vi "Control.vi"(4 "vB":fxp<+,28,8>, 5 "vB_o":fxp<+,28,8>, 6 "Vb":fxp<+,27,7>, 7 "e(k-1)":fxp<+/-,29,9>, 8 "s_c":bool, 9 "Io":fxp<+/-,25,5>, 10 "u(k-1)":fxp<+,20,0>, 11 "v_ref":fxp<+,28,8>) -> (2 "u(k)":fxp<+,20,0>, 3 "e(k)":fxp<+/-,29,9>)   [LabVIEW 2015]
uses:
  <vilib>/rvi/FXPMathLib/FxpMul/XNode/nifxpmath_Multiplier.xnode
  <vilib>/rvi/FXPMathLib/FxpSub/XNode/nifxpmath_Sub.xnode
  <vilib>/rvi/FXPMathLib/FxpAdd/XNode/nifxpmath_Add.xnode
  <vilib>/rvi/FXPMathLib/sim/FxpSim.dll
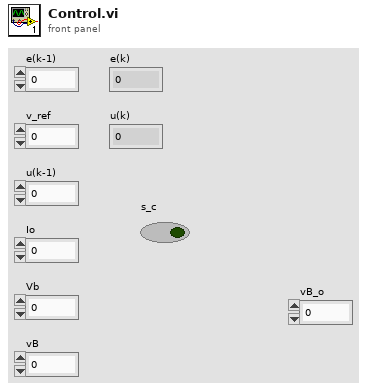
[diagram p1: front panel]
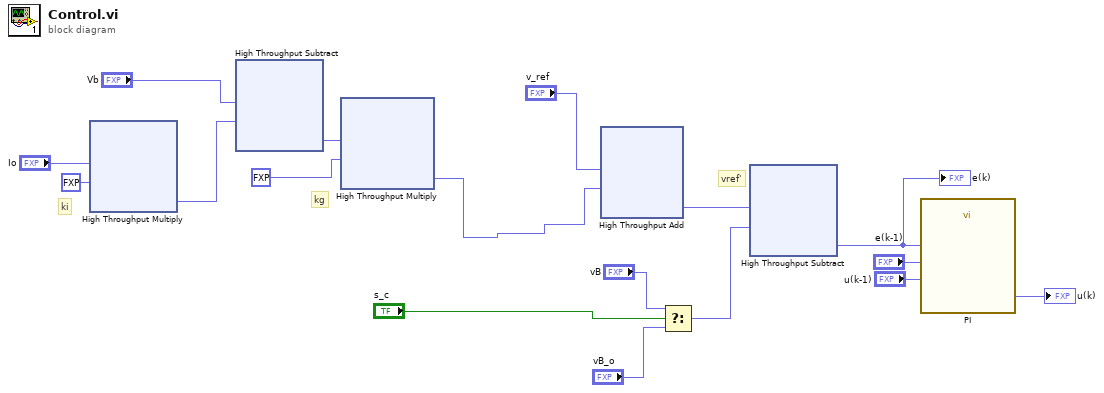
[diagram p0: block diagram]
diagram:
  # "vref'"
  # "kg"
  # "ki"
  n1 = xnode ("High Throughput Multiply")("x"="Io", "y"=fxp<+,3,3> 6.0) -> ("x*y"=w10:fxp<+/-,28,8>)
  n2 = xnode "High Throughput Subtract"("x"="Vb", "y"=w10) -> ("x-y"=w11:fxp<+/-,29,9>)
  n3 = xnode ("High Throughput Multiply")("x"=w11, "y"=fxp<+,2,2> 2.0) -> ("x*y"=w1:fxp<+/-,31,11>)
  n4 = xnode ("High Throughput Add")("x"="v_ref", "y"=w1) -> ("x+y"=w14:fxp<+,28,8>)
  n5 = Select(t="vB", s="s_c", f="vB_o") -> (s? t:f=w3:fxp<+,28,8>)
  n6 = xnode "High Throughput Subtract"("x"=w14, "y"=w3) -> ("x-y"=w15:fxp<+/-,29,9>)
  "e(k)" <- w15
  n7 = call "PI.vi"("u(k-1)_in"="u(k-1)", "e(k-1)_in"="e(k-1)", "e(k)_in"=w15) -> ("u(k)_in"=→"u(k)":fxp<+,20,0>)  [unwired: 8 in]
